vi "CollectQueueLoop.vi"(0 "reference in":refnum<class "DAQ_Base.lvclass">, 5 "error in (no error)":errorcluster) -> (14 "reference out":refnum<class "DAQ_Base.lvclass">, 19 "error out":errorcluster)   [LabVIEW 2020, in "DAQ.lvlib" / "DAQ_Base.lvclass"]
uses:
  DAQ_Base.lvclass
  E:/01_Project/CXXXX/GKN/C18726_27program_191115004/software/DAQ/DAQ_operation_type.ctl
panel:
  out "波形图":dbl[][](graph)
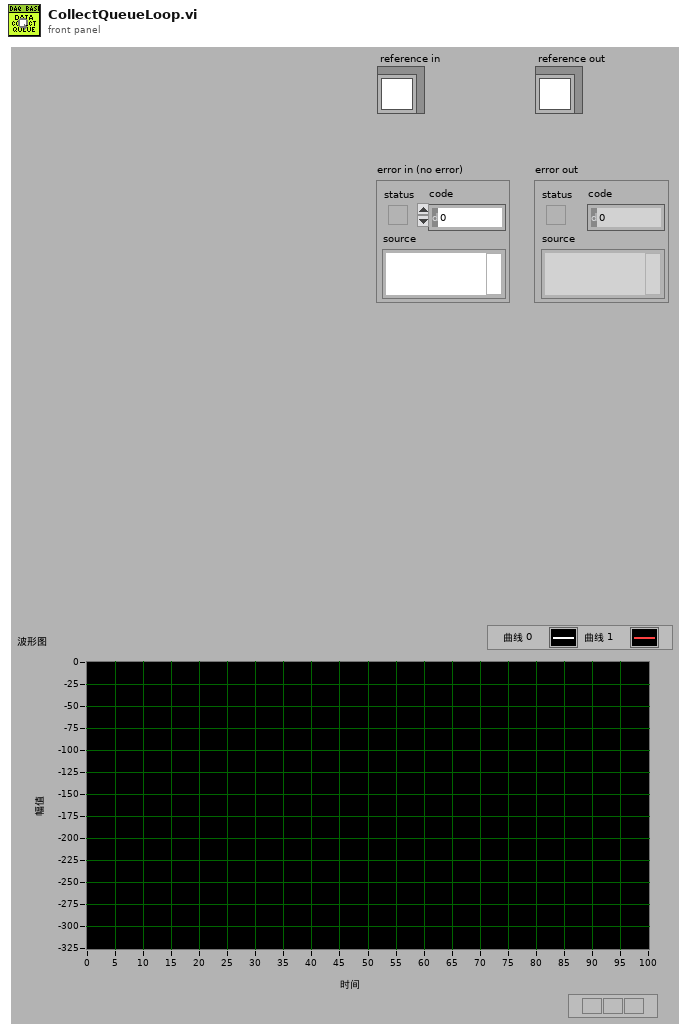
[diagram p1: front panel]
types:
  T1 = typedef "DAQ_operation_type.ctl" = enum16{"idle", "read", "write", "clear", "init", "destroy"}
  T2 = typedef "DAQ.lvlib/DAQ_Base.lvclass/ObjectAttributesRef.ctl" = refnum<data-value>
  T3 = typedef "DAQ.lvlib/DAQ_Base.lvclass/ObjectAttributes.ctl" = cluster{"MyAttribute":dbl, "RootPath":path, "DAQSettings":T4, "DaqCollector":cluster{"CollectDataQueue":refnum<queue>, "ArryDataCollectorChannel":T10[], "RealTimeValues":dbl[]}, "CollectorChannelEnable":bool[]}
  T4 = typedef "DAQ.lvlib/DAQ_Base.lvclass/DAQSettings.ctl" = cluster{"SampleSettings":T5, "AI_ChannelSettings":T6, "AO_ChannelSettings":T8, "Cnt_ChannelSettings":T9}
  T5 = typedef "DAQ.lvlib/DAQ_Base.lvclass/SampleSettings.ctl" = cluster{"samples per channel":i32, "SampleRate":dbl, "TansMaxLength":dbl, "ReadTimeOut":dbl, "时钟源":tag}
  T6 = typedef "DAQ.lvlib/DAQ_Base.lvclass/AI_ChannelSettings.ctl" = cluster{"AI_SettingsArry":cluster{"DeviceName":tag, "physical channels":tag, "AssignName":string, "输入信号类型":T7, "Max_value":dbl, "Min_value":dbl, "单位":i32, "shunt resistor location":i32, "external shunt resistor value":dbl, "标定系数":cluster{"Scale":dbl, "Offset":dbl}}[]}
  T7 = typedef "AI信号类型.ctl" = i32
  T8 = typedef "DAQ.lvlib/DAQ_Base.lvclass/AO_ChannelSettings.ctl" = cluster{"布尔":bool}
  T9 = typedef "DAQ.lvlib/DAQ_Base.lvclass/Cnt_ChannelSettings.ctl" = cluster{"Cnt_ChannelSettings":cluster{"类型":enum16{"Linear", "Rotate"}, "CounterNbr":tag, "AssignName":string, "单位":u16, "decoding type":u16, "PPR_DistancePerPulse":dbl, "Initial Position ":dbl, "z index enable":bool, "z index phase":i32, "source":tag}[]}
  T10 = typedef "DAQ.lvlib/DAQ_Base.lvclass/DataCollector.ctl" = cluster{"DataCollectArry":dbl[][], "Update":bool}
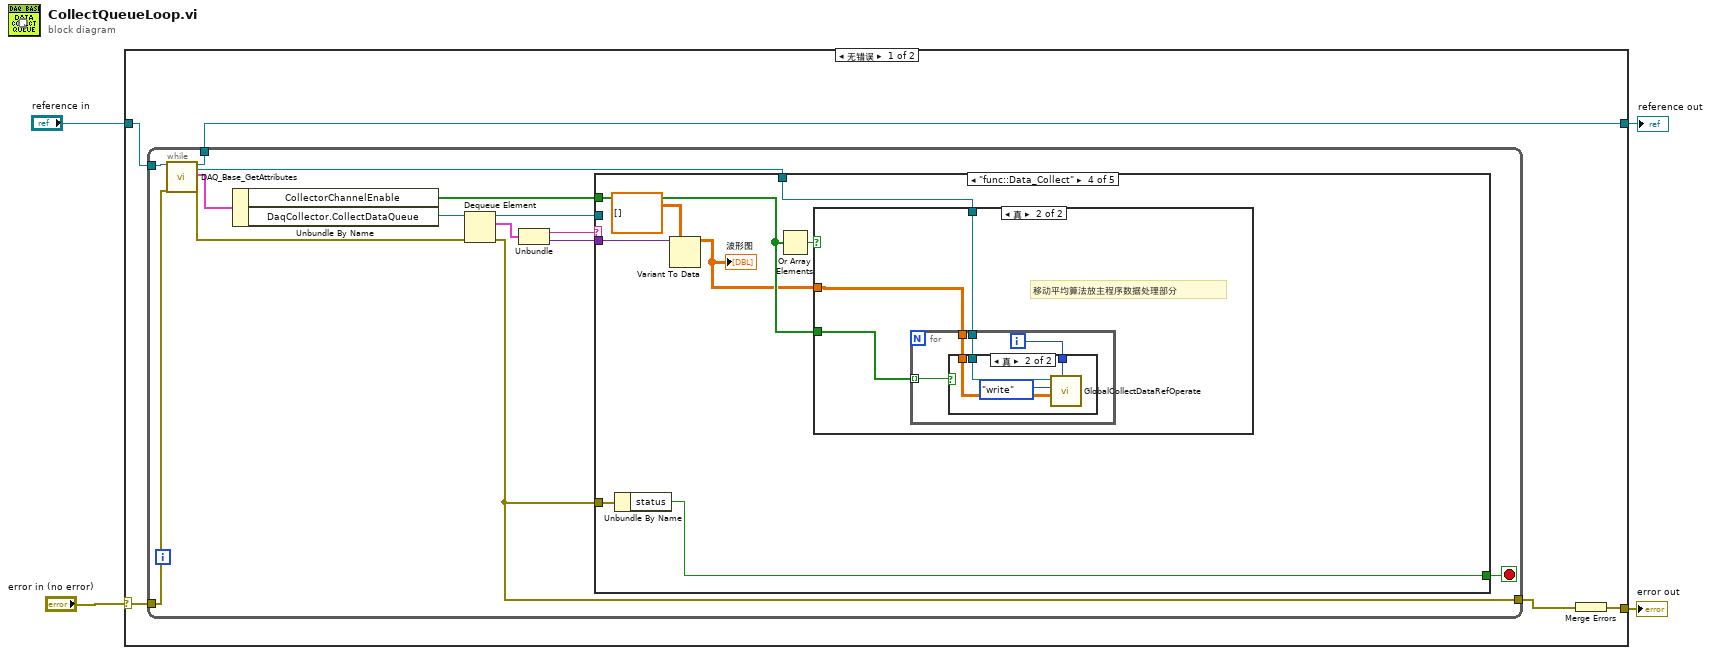
[diagram p0: block diagram]
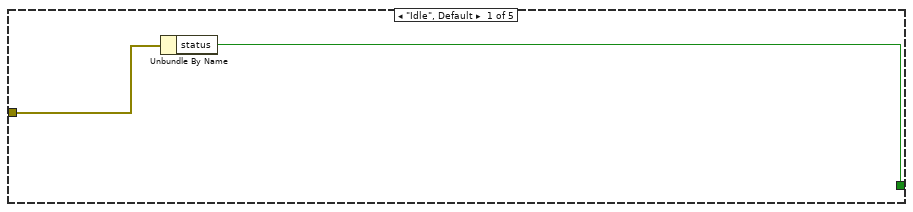
[diagram p2: hidden frame]
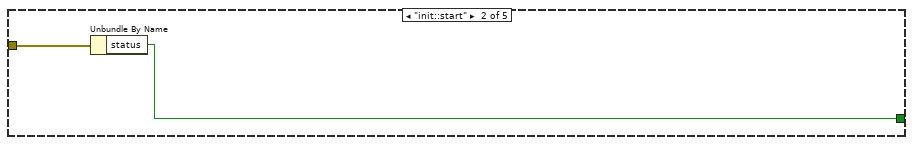
[diagram p3: hidden frame]
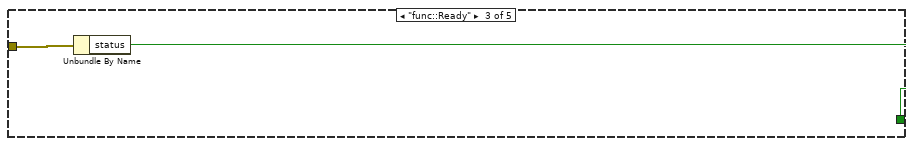
[diagram p4: hidden frame]
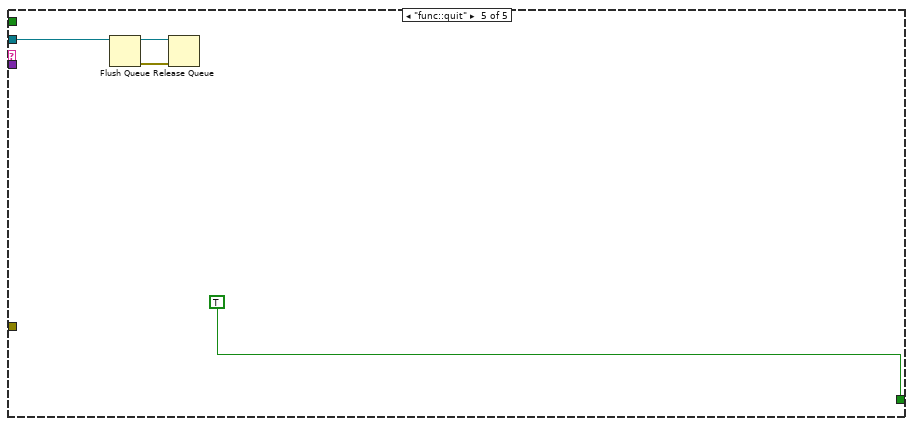
[diagram p7: hidden frame]
diagram:
  n1 = case shown="无错误" "error in (no error)" {
    selector: "error in (no error)" -> [w6 w54]
    tunnel: [w9 w54] -> w3
    tunnel: [w5 w53] -> w1
    tunnel: "reference in" -> [w7 w53]
    frame No Error {
      n2 = while {
        tunnel: [w18] -> w8
        tunnel: w7 -> [w15]
        tunnel: w6 -> [w14]
        tunnel: [w13] -> w5
        stop <- w23 stop-if-true
        n3 = call "DAQ_Base_GetAttributes.vi"("reference in"=w15, "error in (no error)"=w14) -> ("reference out"=w13:refnum<class "DAQ_Base.lvclass">, "attributes ref"=w12:T2, "attributes"=w11:T3, "error out"=w10:errorcluster)  [unwired: 14 in]
        n4 = Unbundle By Name(w11) -> ("CollectorChannelEnable"=w17:bool[], "DaqCollector.CollectDataQueue"=w16:refnum<queue>)
        n5 = Dequeue Element(queue=w16, error in (no error)=w10) -> (queue out=w19:refnum<queue>, element=w22:cluster{string, "Variant":variant}, error out=w18:errorcluster)  [unwired: 1 in, 1 out]
        n6 = Unbundle(w22) -> (w21:string, "Variant"=w20:variant)
        n7 = case shown="\"func::Data_Collect\"" w21 {
          tunnel: w20 -> [_ _ _ w37 _]
          tunnel: w19 -> [_ _ _ _ w50]
          tunnel: [w24 w26 w28 w35 TRUE] -> w23
          tunnel: w18 -> [w25 w27 w29 w36 _]
          tunnel: w17 -> [_ _ _ w32 _]
          tunnel: w12 -> [_ _ _ w30 _]
          frame "Idle", Default {
            n8 = Unbundle By Name(w25) -> ("status"=w24:bool)
          }
          frame "init::start" {
            n9 = Unbundle By Name(w27) -> ("status"=w26:bool)
          }
          frame "func::Ready" {
            n10 = Unbundle By Name(w29) -> ("status"=w28:bool)
          }
          frame "func::Data_Collect" {
            n11 = Unbundle By Name(w36) -> ("status"=w35:bool)
            n12 = Variant To Data(type=dbl[][] [] ("波形图"), Variant=w37) -> (data=w31:dbl[][])  [unwired: 1 in, 1 out]
            "波形图" <- w31
            n13 = Or Array Elements(Boolean array=w32) -> (logical OR=w33:bool)
            n14 = case shown="真" w33 {
              tunnel: w31 -> [_ w40]
              tunnel: w32 -> [_ w38]
              tunnel: w30 -> [_ w39]
              frame False {
              }
              frame True {
                # "移动平均算法放主程序数据处理部分"
                n15 = for {
                  tunnel: w40 -> [w44]
                  tunnel: w39 -> [w43]
                  tunnel: w38 -> [w41] mode=indexing
                  i -> [w42]
                  n16 = case shown="真" w41 {
                    tunnel: w44 -> [_ w48]
                    tunnel: w43 -> [_ w47]
                    tunnel: w42 -> [_ w45]
                    frame False {
                    }
                    frame True {
                      n17 = call "GlobalCollectDataRefOperate.vi"("ChannelNbr"=w45, "DatIn"=w48, "operation"=DAQ_operation_type."write" ("opearte"), "attributes ref"=w47) -> ()  [unwired: 5 in, 3 out]
                    }
                  }
                }
              }
            }
          }
          frame "func::quit" {
            n18 = Flush Queue(queue=w50) -> (queue out=w51:refnum<queue>, error out=w52:errorcluster)  [unwired: 1 in, 1 out]
            n19 = Release Queue(queue=w51, error in (no error)=w52) -> ()  [unwired: 1 in, 3 out]
          }
        }
      }
      n20 = Merge Errors(w8) -> (w9:errorcluster)
    }
    frame Error {
    }
  }
  "error out" <- w3
  "reference out" <- w1
